vi "Hatch2VerCol.vi"(8 "Color Off":T2={"Alpha"=1.0, "Color"=0} {"Alpha" min=0.0 max=1.0 scale=0.0..1.0}, 9 "Color On":T2={"Alpha"=1.0, "Color"=0} {"Alpha" min=0.0 max=1.0 scale=0.0..1.0}, 10 "Z":dbl, 11 "Path":T4) -> (1 "Normals":T1[](array[typedef]), 2 "Colors":cluster{"R":sgl, "G":sgl, "B":sgl, "A":sgl}[](array[cluster]), 3 "VertexArray3d":T1[](array[typedef]))   [LabVIEW 2014]
uses:
  TypeDefs/Point2D.ctl
  TypeDefs/Point3D.ctl
  TypeDefs/Color.ctl
  <vilib>/picture/3D Picture Control/NI_3D Picture Control.lvlib
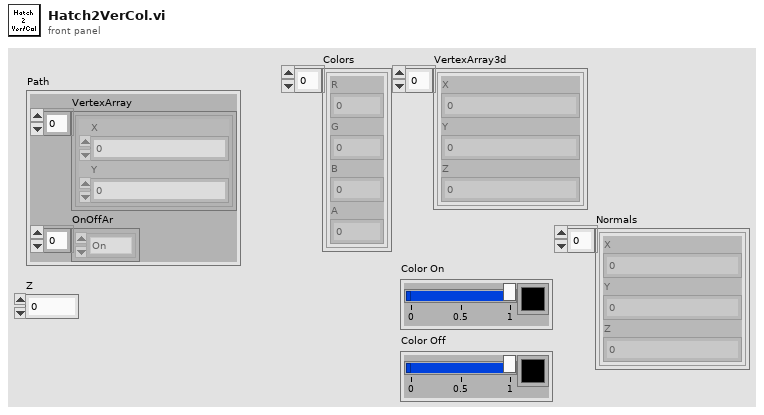
[diagram p1: front panel]
types:
  T1 = typedef "Point3D.ctl" = cluster{"X":sgl, "Y":sgl, "Z":sgl}
  T2 = typedef "Color.ctl" = cluster{"Alpha":dbl, "Color":u32}
  T3 = typedef "Point2D.ctl" = cluster{"X":sgl, "Y":sgl}
  T4 = cluster{"VertexArray":T3[], "OnOffAr":enum16{"On", "Off"}[]}
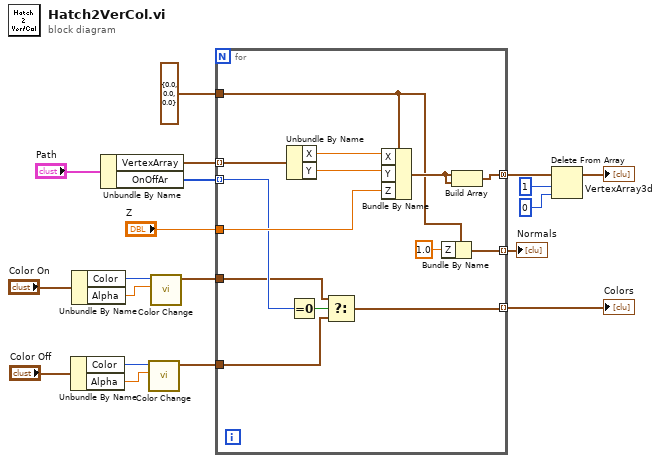
[diagram p0: block diagram]
diagram:
  n1 = Unbundle By Name("Color Off") -> ("Color"=w7:u32, "Alpha"=w6:dbl)
  n2 = Unbundle By Name("Color On") -> ("Color"=w10:u32, "Alpha"=w9:dbl)
  n3 = Unbundle By Name("Path") -> ("VertexArray"=w18:T3[], "OnOffAr"=w17:enum16{"On", "Off"}[])
  n4 = call <vilib>:"Color Change.vi"("Alpha"=w6, "Color"=w7) -> ("RGBA"=w14:cluster{"R":sgl, "G":sgl, "B":sgl, "A":sgl})  [unwired: 9 in]
  n5 = call <vilib>:"Color Change.vi"("Alpha"=w9, "Color"=w10) -> ("RGBA"=w15:cluster{"R":sgl, "G":sgl, "B":sgl, "A":sgl})  [unwired: 9 in]
  n6 = for {
    tunnel: w18 -> [w33] mode=indexing
    tunnel: w17 -> [w28] mode=indexing
    tunnel: "Z" -> [w30]
    tunnel: w15 -> [w27]
    tunnel: w14 -> [w26]
    tunnel: T1 {"X"=0.0, "Y"=0.0, "Z"=0.0} ("Point3D") -> [w22]
    tunnel: [w24] -> w5 mode=concatenating
    tunnel: [w23] -> w12 mode=indexing
    tunnel: [w20] -> w1 mode=indexing
    n7 = Unbundle By Name(w33) -> ("X"=w32:sgl, "Y"=w31:sgl)
    n8 = Equal To 0?(x=w28) -> (x = 0?=w29:bool)
    n9 = Select(t=w27, s=w29, f=w26) -> (s? t:f=w23:cluster{"R":sgl, "G":sgl, "B":sgl, "A":sgl})
    n10 = Bundle By Name(cluster=w22, "X"=w32, "Y"=w31, "Z"=w30) -> (w25:T1)
    n11 = Bundle By Name(cluster=w22, "Z"=sgl 1.0) -> (w20:T1)
    n12 = Build Array(w25, w25) -> (w24:T1[])
  }
  "Colors" <- w12
  "Normals" <- w1
  n13 = Delete From Array(array=w5, length=1, index=0) -> (array with subset deleted=→"VertexArray3d":T1[])  [unwired: 1 out]
